vi "Fuzzy logic.vi"(4 "Floor height":dbl=3.0, 6 "Time per stop":i32=5, 7 "Fuzzy system path":path, 8 "Time per floor":i32=2, 9 "Elevator states array":T1[](array[typedef]), 11 "Floors to serve":cluster{"H call":dbl, "Up":bool}[](array[cluster])) -> (1 "Elevator states array out":T1[](array[typedef]), 3 "Floors to serve out":cluster{"H call":dbl, "Up":bool}[](array[cluster]))   [LabVIEW 2019]
uses:
  Type defs/Elevator states.ctl
  Type defs/Elevator position.ctl
  Type defs/Car buttons.ctl
  <vilib>/addons/Fuzzy Logic/FL Fuzzy Controller (MISO).vi
  <vilib>/addons/Fuzzy Logic/NI_Fuzzy_Logic_API.lvlib
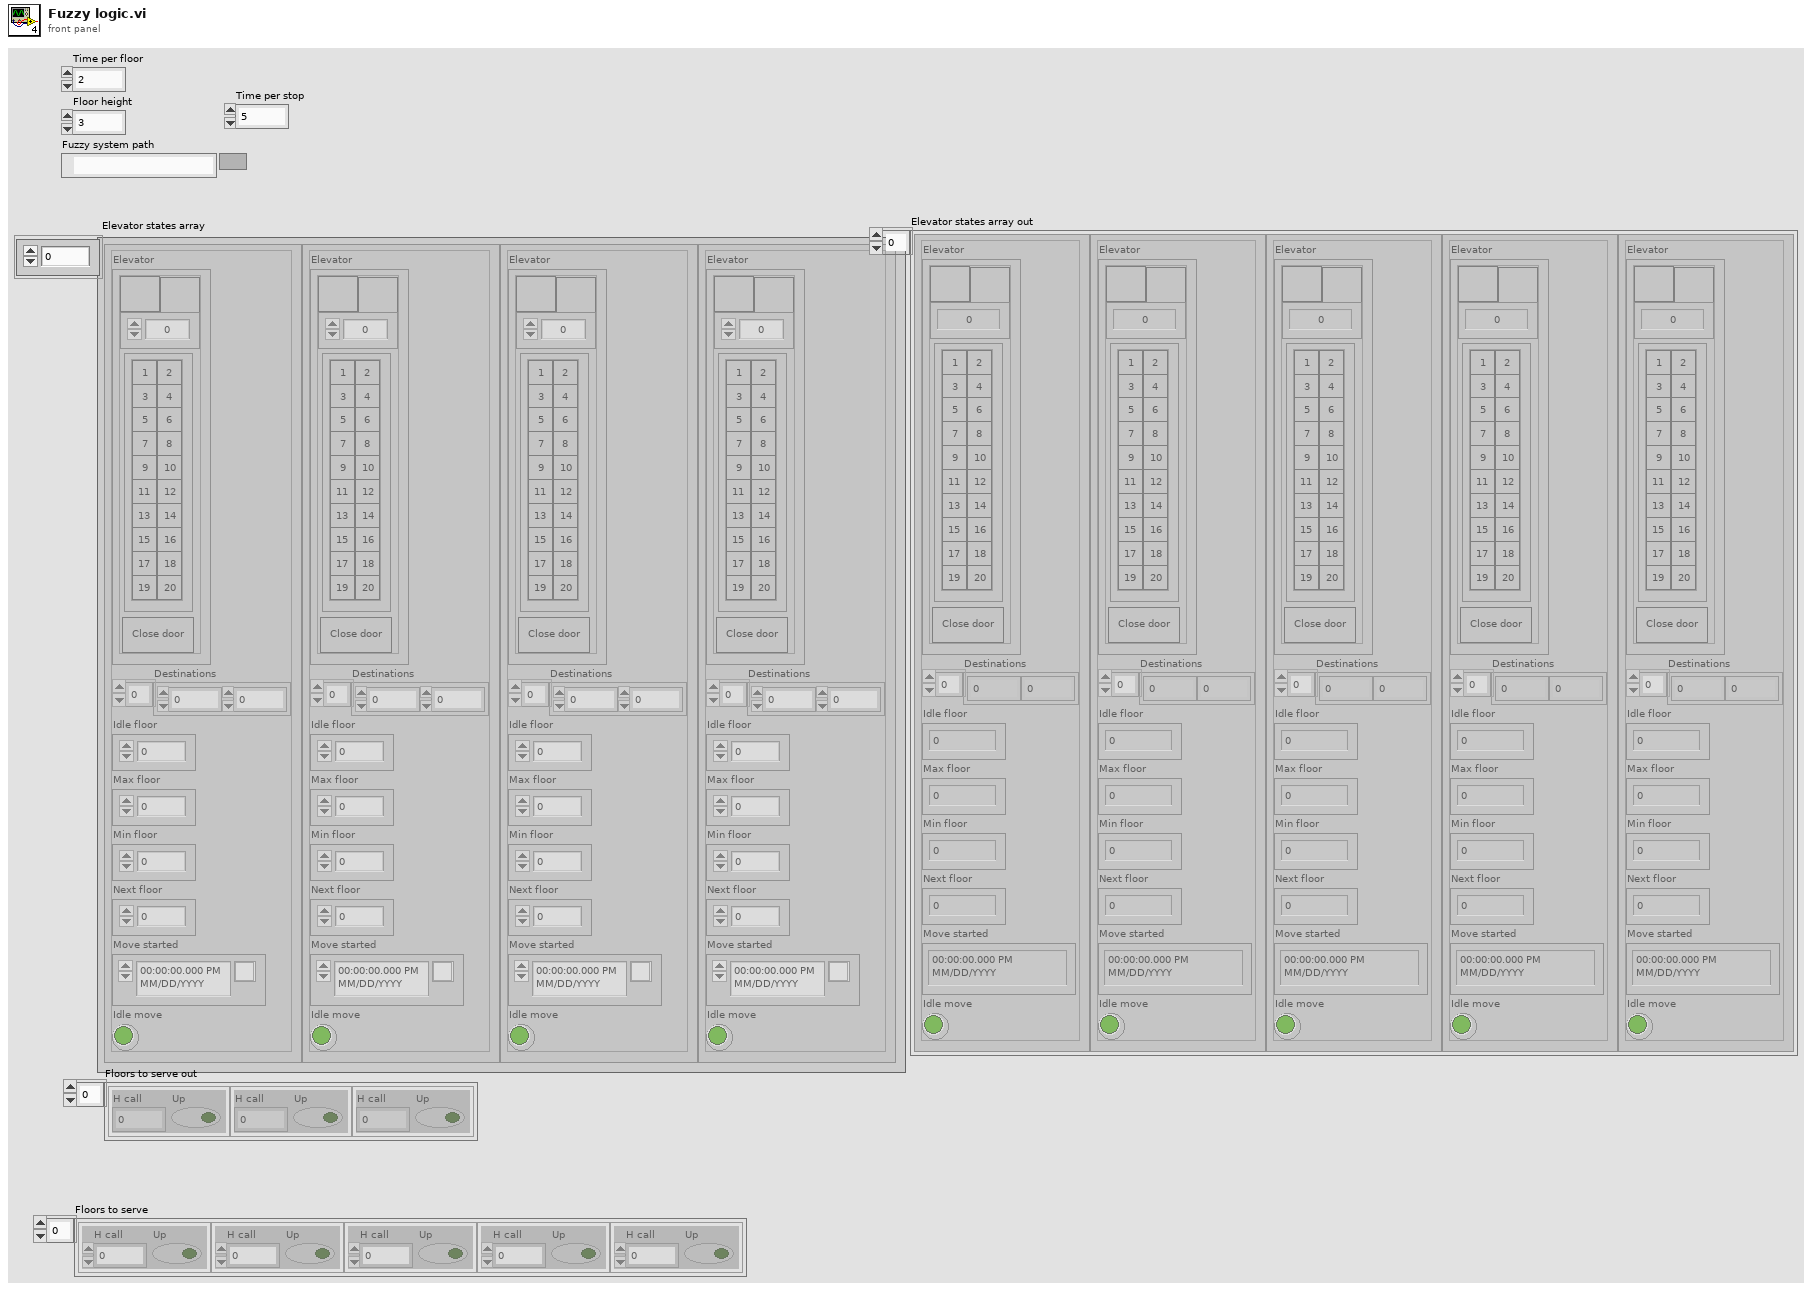
[diagram p1: front panel]
types:
  T1 = typedef "Elevator states.ctl" = cluster{"Elevator":T2, "Destinations":i32[], "Idle floor":u16, "Max floor":u16, "Min floor":u16, "Next floor":u16, "Move started":timestamp, "Idle move":bool}
  T2 = typedef "Elevator position.ctl" = cluster{"Up Button":bool, "Current floor":u16, "Down Button":bool, "Car":T3, "Close door":bool}
  T3 = typedef "Car buttons.ctl" = cluster{"Blank Button":bool, "Blank Button 2":bool, "Blank Button 3":bool, "Blank Button 4":bool, "Blank Button 5":bool, "Blank Button 6":bool, "Blank Button 7":bool, "Blank Button 8":bool, "Blank Button 9":bool, "Blank Button 10":bool, "Blank Button 11":bool, "Blank Button 12":bool, "Blank Button 13":bool, "Blank Button 14":bool, "Blank Button 15":bool, "Blank Button 16":bool, "Blank Button 17":bool, "Blank Button 18":bool, "Blank Button 19":bool, "Blank Button 20":bool}
  T4 = typedef "NI_Fuzzy_Logic_API.lvlib/FL System.ctl" = cluster{"input variables":T5[], "output variables":T5[], "rules":T8[], "defuzzification method":T14, "description":string, "user MF interpolating polynomials":T15[]}
  T5 = typedef "NI_Fuzzy_Logic_API.lvlib/FL Variable.ctl" = cluster{"name":string, "range":dbl[], "MFs":T6[]}
  T6 = typedef "NI_Fuzzy_Logic_API.lvlib/FL Membership Function.ctl" = cluster{"name":string, "shape":T7, "points":dbl[], "color":u32, "user-defined shape index":i32}
  T7 = typedef "NI_Fuzzy_Logic_API.lvlib/FL Membership Function Shape.ctl" = u16
  T8 = typedef "NI_Fuzzy_Logic_API.lvlib/FL Rule.ctl" = cluster{"antecedents":T9[], "antecedent connective":T11, "consequents":T12[], "consequent implication":T13, "degree of support":dbl}
  T9 = typedef "NI_Fuzzy_Logic_API.lvlib/FL Antecedent.ctl" = cluster{"Var Index":i32, "MF Index":i32, "Cond":T10}
  T10 = typedef "NI_Fuzzy_Logic_API.lvlib/FL Modifier.ctl" = u16
  T11 = typedef "NI_Fuzzy_Logic_API.lvlib/FL Antecedent Connective.ctl" = u16
  T12 = typedef "NI_Fuzzy_Logic_API.lvlib/FL Consequent.ctl" = cluster{"Var Index":i32, "MF Index":i32, "Cond":T10}
  T13 = typedef "NI_Fuzzy_Logic_API.lvlib/FL Consequent Implication.ctl" = u16
  T14 = typedef "NI_Fuzzy_Logic_API.lvlib/FL Defuzzification.ctl" = u16
  T15 = typedef "NI_Fuzzy_Logic_API.lvlib/FL Interpolating polynomials.ctl" = cluster{"X":dbl[], "Y":dbl[], "Y(x) coeff":dbl[][], "X(y) coeff":dbl[][], "Area(y) coeff":dbl[][], "coa_x(y) coeff":dbl[][]}
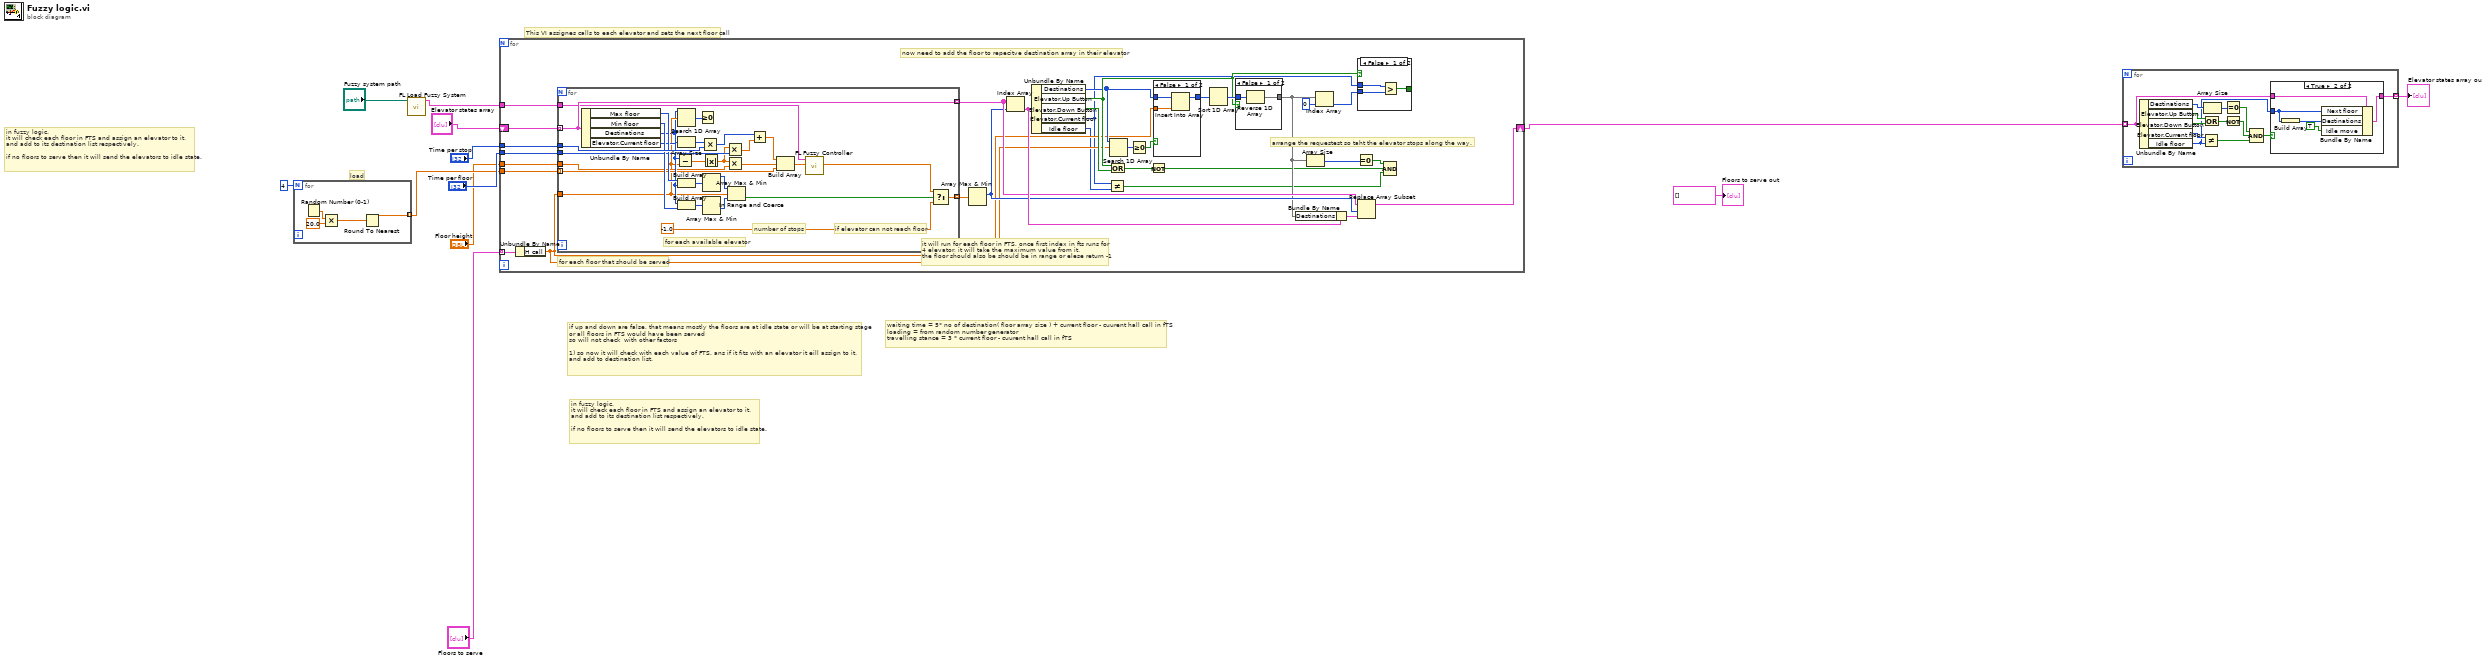
[diagram p0: block diagram]
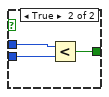
[diagram p3: hidden frame]
diagram:
  # "waiting time = 5* no of destination( floor array size ) + current floor - cuurent hall call in fTS\nloading = from random number generator\ntravelling stance = 3 * current floor - cuurent hall call in fTS"
  # "in fuzzy logic.\nit will check each floor in FTS and assign an elevator to it.\nand add to its destination list respectively.\n\nif no floors to serve then it will send the elevators to idle state."
  # "in fuzzy logic.\nit will check each floor in FTS and assign an elevator to it.\nand add to its destination list respectively.\n\nif no floors to serve then it will send the elevators to idle state."
  # "if up and down are false, that means mostly the floors are at idle state or will be at starting stage\nor all floors in FTS would have been served\nso will not check  with other factors\n\n1) so now it will check with each value of FTS. ans if it fits with an elevator it eill assign to it.\nand add to destination list."
  # "load"
  # "This VI assignes calls to each elevator and sets the next floor call"
  n1 = for {
    N: 4 -> [_]
    tunnel: [w13] -> w7 mode=indexing
    n2 = Random Number (0-1)() -> (number: 0 to 1=w16:dbl)
    n3 = Multiply(x=w16, y=20.0) -> (x*y=w14:dbl)
    n4 = Round To Nearest(number=w14) -> (nearest integer value=w13:dbl)
  }
  n5 = call <vilib>:"FL Load Fuzzy System.vi"("file path"="Fuzzy system path") -> ("fuzzy system out"=w5:T4)  [unwired: 1 in, 9 out]
  n6 = for {
    tunnel: "Time per stop" -> [w47]
    tunnel: "Floors to serve" -> [w46] mode=indexing
    tunnel: "Time per floor" -> [w45]
    tunnel: w7 -> [w44]
    tunnel: "Floor height" -> [w43]
    tunnel: w5 -> [w42]
    shift-right: [w34] -> w2
    shift-left: "Elevator states array" -> [w35]
    # "now need to add the floor to repecitve destination array in their elevator"
    # "it will run for each floor in FTS, once first index in fts runs for\n4 elevator, it will take the maximum value from it. \nthe floor should also be should be in range or elese return -1"
    # "arrange the requestest so taht the elevator stops along the way."
    # "for each floor that should be served"
    n7 = Unbundle By Name(w46) -> ("H call"=w26:dbl)
    n8 = for {
      tunnel: w35 -> [w88] mode=indexing
      tunnel: [w88] -> w37 mode=indexing
      tunnel: w47 -> [w87]
      tunnel: w26 -> [w63]
      tunnel: w45 -> [w77]
      tunnel: w44 -> [w70] mode=indexing
      tunnel: w43 -> [w75]
      tunnel: w42 -> [w68]
      tunnel: [w64] -> w41 mode=indexing
      # "if elevator can not reach floor"
      # "for each available elevator"
      # "number of stops"
      n9 = Unbundle By Name(w88) -> ("Max floor"=w86:u16, "Min floor"=w83:u16, "Destinations"=w62:i32[], "Elevator.Current floor"=w79:u16)
      n10 = Subtract(x=w79, y=w63) -> (x-y=w78:dbl)
      n11 = Search 1D Array(1D array=w62, element=w63) -> (index of element=w61:i32)  [unwired: 1 in]
      n12 = Array Size(array=w62) -> (size(s)=w80:i32)
      n13 = Build Array(w86, w79) -> (w85:u16[])
      n14 = Build Array(w79, w83) -> (w82:u16[])
      n15 = Greater Or Equal To 0?(x=w61) -> ()  [unwired: 1 out]
      n16 = Multiply(x=w80, y=w87) -> (x*y=w74:i32)
      n17 = Absolute Value(x=w78) -> (abs(x)=w76:dbl)
      n18 = Array Max & Min(array=w85) -> (max value=w84:u16)  [unwired: 3 out]
      n19 = Array Max & Min(array=w82) -> (min value=w81:u16)  [unwired: 3 out]
      n20 = Multiply(x=w76, y=w77) -> (x*y=w73:dbl)
      n21 = Multiply(x=w76, y=w75) -> (x*y=w71:dbl)
      n22 = In Range and Coerce(upper limit=w84, x=w63, lower limit=w81) -> (In Range?=w67:bool)  [unwired: 1 out]
      n23 = Add(x=w74, y=w73) -> (x+y=w72:dbl)
      n24 = Build Array(w72, w71, w70) -> (w69:dbl[])
      n25 = call-poly <vilib>:"FL Fuzzy Controller.vi"("input values"=w69, "fuzzy system in"=w68) -> ("output value"=w66:dbl)  [unwired: 1 in, 8 out]
      n26 = Select(t=w66, s=w67, f=-1.0) -> (s? t:f=w64:dbl)
    }
    n27 = Array Max & Min(array=w41) -> (max index (indices)=w36:i32)  [unwired: 3 out]
    n28 = Index Array(array=w37, index=w36) -> (element=w40:T1)
    n29 = Unbundle By Name(w40) -> ("Destinations"=w27:i32[], "Elevator.Up Button"=w31:bool, "Elevator.Down Button"=w33:bool, "Elevator.Current floor"=w19:u16, "Idle floor"=w17:u16)
    n30 = Not Equal?(x=w19, y=w17) -> (x != y?=w18:bool)
    n31 = Search 1D Array(1D array=w27, element=w26) -> (index of element=w28:i32)  [unwired: 1 in]
    n32 = Compound Arithmetic op=OR(w31, w33) -> (w21:bool)
    n33 = Greater Or Equal To 0?(x=w28) -> (x >= 0?=w25:bool)
    n34 = Not(x=w21) -> (.not. x?=w20:bool)
    n35 = case shown="False" w25 {
      tunnel: [w50 w51] -> w38
      tunnel: w27 -> [w49 w51]
      tunnel: w26 -> [w48 _]
      frame False {
        n36 = Insert Into Array(array=w49, new element=w48) -> (w50:i32[])  [unwired: 1 in]
      }
      frame True {
      }
    }
    n37 = Sort 1D Array(array=w38) -> (sorted array=w39:i32[])
    n38 = case shown="False" w31 {
      tunnel: [w59 w60] -> w24
      tunnel: w39 -> [w58 w60]
      frame False {
        n39 = Reverse 1D Array(array=w58) -> (reversed array=w59:i32[])
      }
      frame True {
      }
    }
    n40 = Bundle By Name(cluster=w40, "Destinations"=w24) -> (w32:T1)
    n41 = Array Size(array=w24) -> (size(s)=w23:i32)
    n42 = Index Array(array=w24, index=0) -> (element=w29:i32)
    n43 = Equal To 0?(x=w23) -> (x = 0?=w22:bool)
    n44 = case shown="False" w31 {
      tunnel: w19 -> [w54 w57]
      tunnel: w29 -> [w53 w56]
      tunnel: [w52 w55] -> _
      frame False {
        n45 = Greater?(x=w54, y=w53) -> (0:w52:bool)
      }
      frame True {
        n46 = Less?(x=w57, y=w56) -> (x < y?=w55:bool)
      }
    }
    n47 = Replace Array Subset(array=w37, new element=w32, index=w36) -> (w34:T1[])
    n48 = Compound Arithmetic op=AND(w22, w20, w18) -> ()  [unwired: 1 out]
  }
  n49 = for {
    tunnel: w2 -> [w90] mode=indexing
    tunnel: [w89] -> w1 mode=indexing
    n50 = Unbundle By Name(w90) -> ("Destinations"=w95:i32[], "Elevator.Up Button"=w100:bool, "Elevator.Down Button"=w99:bool, "Elevator.Current floor"=w98:u16, "Idle floor"=w91:u16)
    n51 = Not Equal?(x=w98, y=w91) -> (x != y?=w93:bool)
    n52 = Array Size(array=w95) -> (size(s)=w97:i32)
    n53 = Compound Arithmetic op=OR(w100, w99) -> (w101:bool)
    n54 = Equal To 0?(x=w97) -> (x = 0?=w96:bool)
    n55 = Not(x=w101) -> (.not. x?=w94:bool)
    n56 = Compound Arithmetic op=AND(w96, w94, w93) -> (w92:bool)
    n57 = case shown="True" w92 {
      tunnel: w91 -> [_ w106]
      tunnel: w90 -> [w102 w105]
      tunnel: [w102 w104] -> w89
      frame False {
      }
      frame True {
        n58 = Build Array(w106) -> (w107:u16[])
        n59 = Bundle By Name(cluster=w105, "Next floor"=w106, "Destinations"=w107, "Idle move"=TRUE) -> (w104:T1)
      }
    }
  }
  "Elevator states array out" <- w1
  "Floors to serve out" <- cluster{"H call":dbl, "Up":bool}[] [] ("Floors to serve out")
